vi "docs--rules.vi"() -> ()   [LabVIEW 2021]
panel:
  in  "Tab Control":T1(tab)
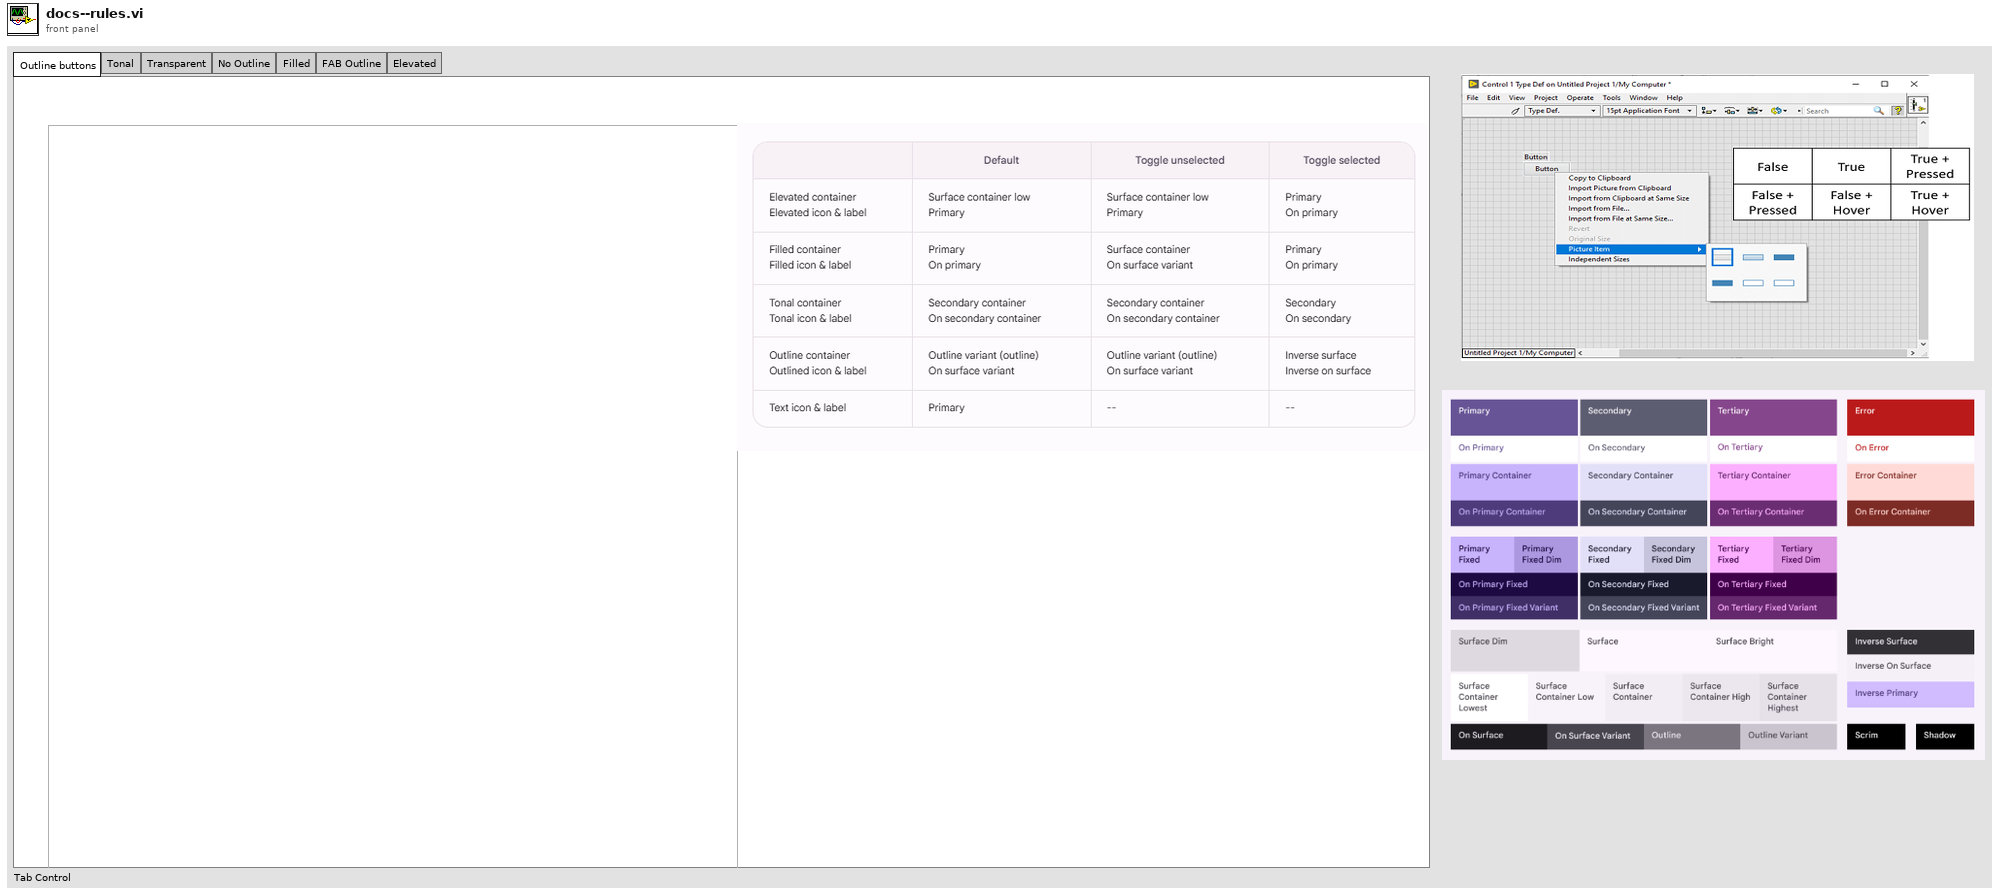
[diagram p1: front panel]
types:
  T1 = enum32{"Outline buttons", "Tonal", "Transparent", "No Outline", "Filled", "FAB Outline", "Elevated"}
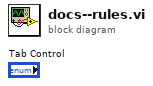
[diagram p0: block diagram]
diagram:
